vi "CE14 Close Connection (SubVI).vi"(8 "error in (no error)":errorcluster, 11 "VISA Refnum in":refnum<visa-resource-name>) -> (0 "error out":errorcluster)   [LabVIEW 2018, in "CE14_eMIC.lvlib"]
uses:
  CE14_eMIC.lvlib
panel:
  in  "milliseconds to wait(100 ms)":u32=100
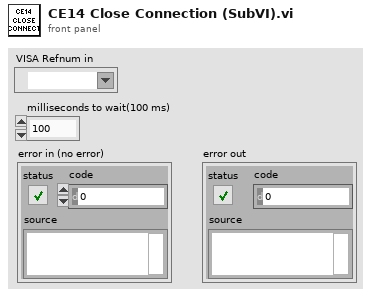
[diagram p1: front panel]
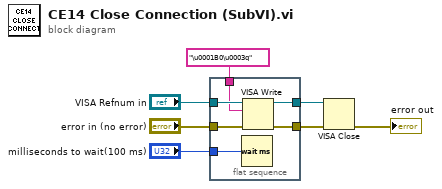
[diagram p0: block diagram]
diagram:
  n1 = flat-sequence {
    tunnel: [w13] -> w7
    tunnel: [w12] -> w1
    tunnel: "VISA Refnum in" -> [w11]
    tunnel: "error in (no error)" -> [w10]
    tunnel: "\u0001B0\u0003q" -> [w9]
    tunnel: "milliseconds to wait(100 ms)" -> [w8]
    frame #0 {
      n2 = Wait (ms)(milliseconds to wait=w8) -> ()  [unwired: 1 out]
      n3 = VISA Write(VISA resource name=w11, write buffer=w9, error in (no error)=w10) -> (VISA resource name out=w12:refnum<visa-resource-name>, error out=w13:errorcluster)  [unwired: 1 out]
    }
  }
  n4 = VISA Close(VISA resource name=w1, error in (no error)=w7) -> (error out=→"error out":errorcluster)
